vi "LV SCISDK Get Parameter String.vi"(8 "error in (no error)":errorcluster, 10 "handle":u64, 11 "Path":string) -> (0 "error out":errorcluster, 1 "function return":i32, 2 "handle out":u64, 3 "value":string)   [LabVIEW 2021, in "SciSDK_Labview.lvlib"]
doc: "SCISDKLABVIEW_DLL_API int LV_SCISDK_GetParameterString(char* Path, char* value, void* handle);"
uses:
  SciSDK_Labview.lvlib
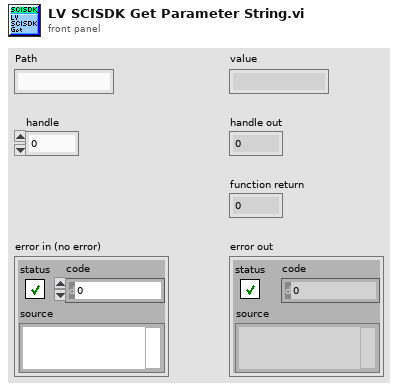
[diagram p1: front panel]
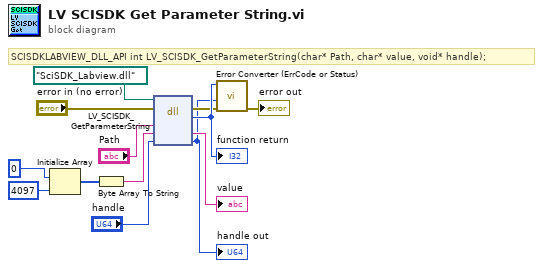
[diagram p0: block diagram]
diagram:
  # "SCISDKLABVIEW_DLL_API int LV_SCISDK_GetParameterString(char* Path, char* value, void* handle);"
  n1 = Initialize Array(u8 0 ("element"), 4097 ("dimension size")) -> (w11:u8[])
  n2 = Byte Array To String(unsigned byte array=w11) -> (string=w10:string)
  n3 = dll-call lib="C:/git/scisdk/SciSDK_VC++/x64/Debug/SciSDK_Labview.dll" fn="LV_SCISDK_GetParameterString"(path in=path "SciSDK_Labview.dll", error in="error in (no error)", "Path"="Path", "value"=w10, "handle"="handle") -> (error out=w4:errorcluster, "return type"=w13:i32, "value"=→"value":string, "handle"=w1:u64)  [unwired: 2 in, 1 out]
  "function return" <- w13
  "handle out" <- w1
  n4 = call "Error Converter (ErrCode or Status).vi"("error in (no error)"=w4, "handle"=w1, "error code"=w13) -> ("error out"=→"error out":errorcluster)  [unwired: 8 in]
